vi "read_TestPoint.vi"() -> ()   [LabVIEW 2014]
panel:
  out "Dup Aardvark Handle":i32
  out "Test Point Val (V)":dbl
  out "error out":errorcluster
  in  "error in (no error)":errorcluster
  in  "Address (0x50)":u16=80 max=1023 format="%.0x"
  in  "Aardvark Handle":i32 min=0
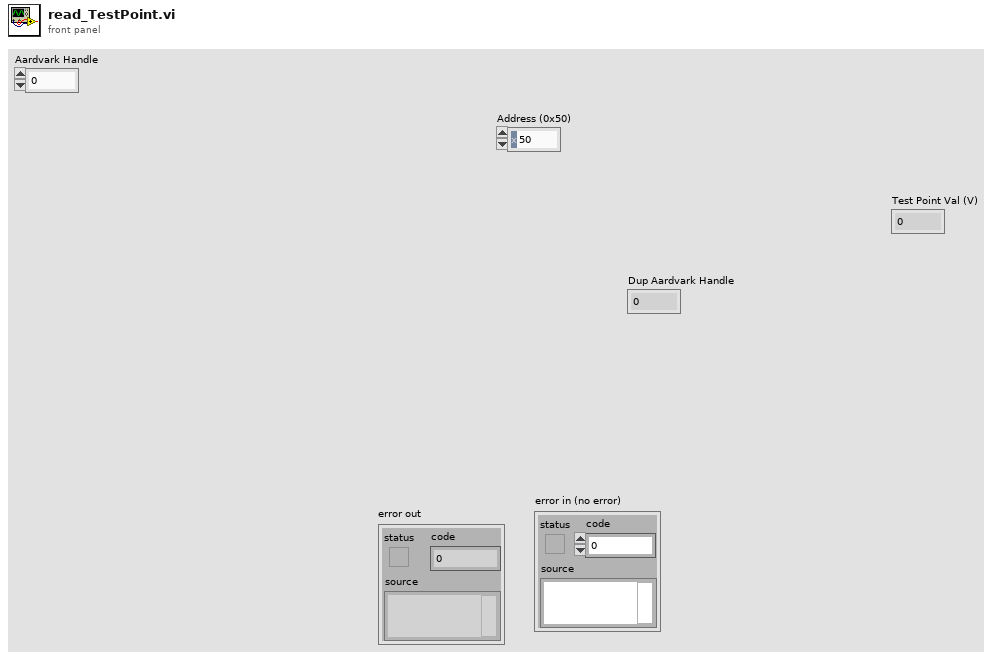
[diagram p1: front panel]
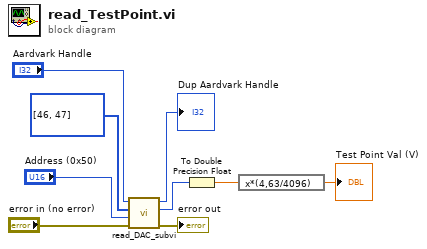
[diagram p0: block diagram]
diagram:
  n1 = call "read_DAC_subvi.vi"("error in (no error)"="error in (no error)", "Address (0x50)"="Address (0x50)", "DAC_ADD"=u8[] [46, 47], "Aardvark Handle"="Aardvark Handle") -> ("error out"=→"error out":errorcluster, "DAC Val"=w2:u16, "Dup Aardvark Handle"=→"Dup Aardvark Handle":i32)  [unwired: 3 in]
  n2 = To Double Precision Float(number=w2) -> (double precision float=w9:dbl)
  n3 = expression code="x*(4,63/4096)"(w9) -> (→"Test Point Val (V)":dbl)
